vi "Logger_Init.vi"(0 "object in":refnum<class "Logger.lvclass">, 5 "error in (no error)":errorcluster) -> (14 "object out":refnum<class "Logger.lvclass">, 19 "error out":errorcluster)   [LabVIEW 2024, in "Logger.lvclass"]
uses:
  Logger.lvclass
  Logger.lvclass/Logger.ctl
panel:
  # "Connector Pane"
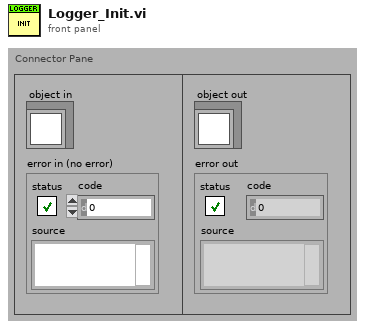
[diagram p1: front panel]
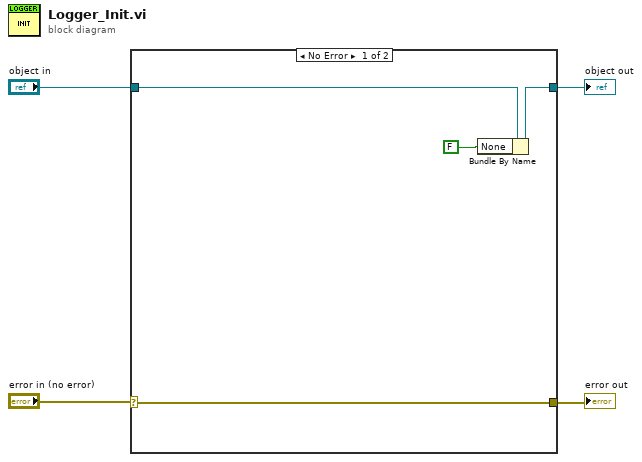
[diagram p0: block diagram]
diagram:
  n1 = case shown="No Error" "error in (no error)" {
    selector: "error in (no error)" -> [w5 w9]
    tunnel: "object in" -> [w8 w10]
    tunnel: [w7 w10] -> w3
    tunnel: [w5 w9] -> w1
    frame No Error {
      n2 = Bundle By Name(cluster=w8, "None"=FALSE) -> (w7:refnum<class "Logger.lvclass">)
    }
    frame Error {
    }
  }
  "object out" <- w3
  "error out" <- w1
